vi "Set Path.vi"(8 "error in (no error)":errorcluster, 10 "Defualt(Sys Relative)":string, 11 "Custom Path":path) -> (0 "error out":errorcluster, 3 "Path":path)   [LabVIEW 2020, in "Logging.lvlib" / "Logger Mananger.lvclass"]
uses:
  Logger Mananger/Logger Mananger.lvclass
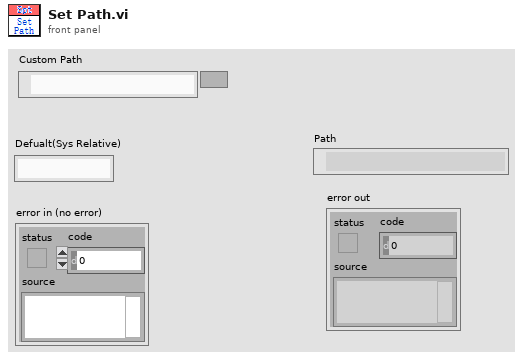
[diagram p1: front panel]
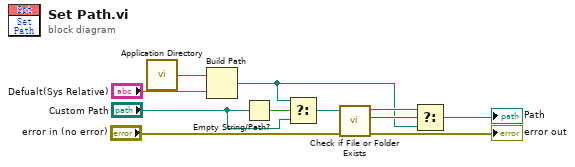
[diagram p0: block diagram]
diagram:
  n1 = call <vilib>:"Application Directory.vi"() -> ("Application Directory"=w11:path)
  n2 = Build Path(base path=w11, name or relative path="Defualt(Sys Relative)") -> (appended path=w3:path)
  n3 = Empty String/Path?(string/path="Custom Path") -> (empty?=w9:bool)
  n4 = Select(t=w3, s=w9, f="Custom Path") -> (s? t:f=w7:path)
  n5 = call <vilib>:"Check if File or Folder Exists.vi"("error in (no error)"="error in (no error)", "path"=w7) -> ("error out"=→"error out":errorcluster, "file or folder exists?"=w6:bool, "dup path"=w5:path)  [unwired: 7 in]
  n6 = Select(t=w5, s=w6, f=w3) -> (s? t:f=→"Path":path)
